vi "Post-Uninstall Custom Action.vi"(10 "Variant":variant) -> (0 "error out":errorcluster)   [LabVIEW 2020]
uses:
  <resource>/dialog/lvconfig.llb/LV Config Read String.vi
  <vilib>/Utility/config.llb/Read Key (String).vi
  <vilib>/Utility/config.llb/Read Key (I32).vi
  <resource>/dialog/lvconfig.llb/LV Config Write String.vi
  <resource>/dialog/lvconfig.llb/LV Config Write Numeric (I32).vi
  <vilib>/Utility/config.llb/NI_LVConfig.lvlib
  <vilib>/zip/NI_Unzip.lvlib
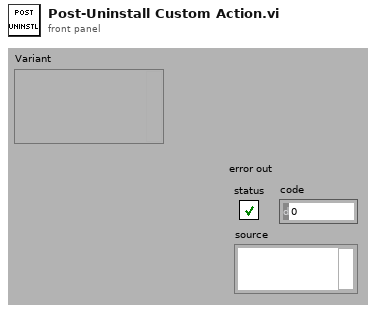
[diagram p1: front panel]
types:
  T1 = typedef "NI_LVConfig.lvlib/Config Data RefNum.ctl" = refnum<k1>
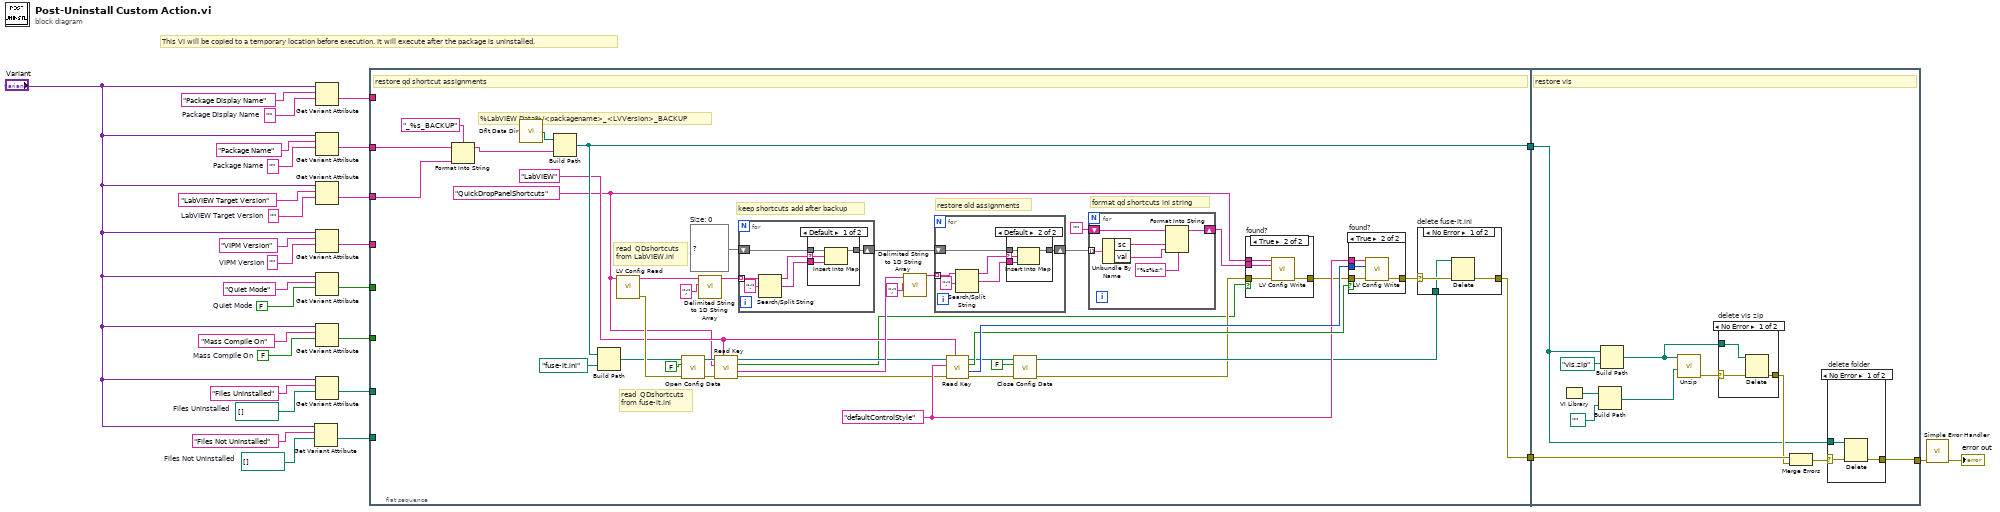
[diagram p0: block diagram]
diagram:
  w5 = path[] []  # Files Not Uninstalled
  w6 = path[] []  # Files Uninstalled
  w12 = FALSE  # Mass Compile On
  w13 = ""  # Package Display Name
  w20 = FALSE  # Quiet Mode
  w23 = ""  # VIPM Version
  w25 = ""  # LabVIEW Target Version
  w27 = ""  # Package Name
  # "This VI will be copied to a temporary location before execution. It will execute after the package is uninstalled."
  n1 = Get Variant Attribute(Variant="Variant", name="Files Not Uninstalled", default value (empty Variant)=w5) -> (value=w10:path[])  [unwired: 1 in, 3 out]
  n2 = Get Variant Attribute(Variant="Variant", name="Package Display Name", default value (empty Variant)=w13) -> (value=w19:string)  [unwired: 1 in, 3 out]
  n3 = Get Variant Attribute(Variant="Variant", name="Package Name", default value (empty Variant)=w27) -> (value=w18:string)  [unwired: 1 in, 3 out]
  n4 = Get Variant Attribute(Variant="Variant", name="LabVIEW Target Version", default value (empty Variant)=w25) -> (value=w17:string)  [unwired: 1 in, 3 out]
  n5 = Get Variant Attribute(Variant="Variant", name="VIPM Version", default value (empty Variant)=w23) -> (value=w16:string)  [unwired: 1 in, 3 out]
  n6 = Get Variant Attribute(Variant="Variant", name="Quiet Mode", default value (empty Variant)=w20) -> (value=w15:bool)  [unwired: 1 in, 3 out]
  n7 = Get Variant Attribute(Variant="Variant", name="Mass Compile On", default value (empty Variant)=w12) -> (value=w14:bool)  [unwired: 1 in, 3 out]
  n8 = Get Variant Attribute(Variant="Variant", name="Files Uninstalled", default value (empty Variant)=w6) -> (value=w9:path[])  [unwired: 1 in, 3 out]
  n9 = flat-sequence {
    tunnel: w19 -> [_]
    tunnel: w18 -> [w32]
    tunnel: w17 -> [w31]
    tunnel: w16 -> [_]
    tunnel: w15 -> [_]
    tunnel: w14 -> [_]
    tunnel: w9 -> [_]
    tunnel: w10 -> [_]
    tunnel: [w65] -> w3
    tunnel: [w62] -> w2
    tunnel: [w114] -> w4
    tunnel: w3 -> [w121]
    tunnel: w2 -> [w111]
    frame #0 {
      w56 = map{string, string} {}  # Size: 0
      w61 = "defaultControlStyle" ("key")
      w42 = "LabVIEW" ("section")
      w39 = "QuickDropPanelShortcuts" ("key")
      # "restore old assignments"
      # "format qd shortcuts ini string"
      # "read  QDshortcuts\nfrom fuse-it.ini"
      # "read  QDshortcuts\nfrom LabVIEW.ini"
      # "keep shortcuts add after backup"
      # "%LabVIEW Data%/<packagename>_<LVVersion>_BACKUP"
      # "restore qd shortcut assignments"
      n10 = Format Into String(format string="_%s_BACKUP", initial string=w32, w31) -> (resulting string=w30:string)  [unwired: 1 in, 1 out]
      n11 = call <vilib>:"Dflt Data Dir.vi"() -> ("App:Default Data Directory"=w68:path)
      n12 = Build Path(base path=w68, name or relative path=w30) -> (appended path=w62:path)
      n13 = Build Path(base path=w62, name or relative path=path "fuse-it.ini") -> (appended path=w41:path)
      n14 = call-poly <resource>:"LV Config Read.vi"("key"=w39) -> ("error out"=w46:errorcluster, "value"=w55:string)  [unwired: 4 in, 1 out]
      n15 = call <vilib>:"Open Config Data.vi"("error in (no error)"=w46, "create file if necessary (T)"=FALSE, "configuration file path"=w41) -> ("error out"=w48:errorcluster, "refnum"=w47:T1)  [unwired: 6 in, 1 out]
      n16 = call <vilib>:"Delimited String to 1D String Array.vi"("delimiter"=";", "delimited string"=w55) -> ("string array"=w57:string[])  [unwired: 9 in]
      n17 = call-poly <vilib>:"Read Key.vi"("section"=w42, "error in (no error)"=w48, "key"=w39, "refnum"=w47) -> ("error out"=w43:errorcluster, "value"=w45:string, "found?"=w36:bool, "refnum out"=w44:T1)  [unwired: 4 in]
      n18 = for {
        tunnel: w57 -> [w78] mode=indexing
        shift-right: [w76] -> w53
        shift-left: w56 -> [w77]
        n19 = Search/Split String(string=w78, search string/char (-)=":") -> (substring before match=w75:string, match + rest of string=w74:string)  [unwired: 1 in, 1 out]
        n20 = case shown="Default" w75 {
          selector: w75 -> [w81 _]
          tunnel: w77 -> [w83 w84]
          tunnel: [w82 w84] -> w76
          tunnel: w74 -> [w80 _]
          frame Default {
            n21 = Insert Into Map(map in=w83, key=w81, value=w80) -> (map out=w82:map{string, string})  [unwired: 2 out]
          }
          frame "" {
          }
        }
      }
      n22 = call <vilib>:"Delimited String to 1D String Array.vi"("delimiter"=";", "delimited string"=w45) -> ("string array"=w52:string[])  [unwired: 9 in]
      n23 = for {
        shift-right: [w90] -> w50
        shift-left: w53 -> [w89]
        tunnel: w52 -> [w87] mode=indexing
        n24 = Search/Split String(string=w87, search string/char (-)=":") -> (substring before match=w86:string, match + rest of string=w85:string)  [unwired: 1 in, 1 out]
        n25 = case shown="Default" w86 {
          selector: w86 -> [_ w93]
          tunnel: [w91 w95] -> w90
          tunnel: w89 -> [w91 w94]
          tunnel: w85 -> [_ w92]
          frame "" {
          }
          frame Default {
            n26 = Insert Into Map(map in=w94, key=w93, value=w92) -> (map out=w95:map{string, string})  [unwired: 2 out]
          }
        }
      }
      n27 = call-poly <vilib>:"Read Key.vi"("section"=w42, "error in (no error)"=w43, "key"=w61, "refnum"=w44) -> ("error out"=w60:errorcluster, "value"=w67:i32, "found?"=w66:bool, "refnum out"=w64:T1)  [unwired: 4 in]
      n28 = call <vilib>:"Close Config Data.vi"("error in (no error)"=w60, "write file if changed (T)"=FALSE, "refnum"=w64) -> ("error out"=w37:errorcluster, "file path"=w40:path)  [unwired: 7 in]
      n29 = for {
        tunnel: w50 -> [w101] mode=indexing
        shift-right: [w96] -> w38
        shift-left: "" -> [w99]
        n30 = Unbundle By Name(w101) -> ("sc"=w98:string, "val"=w97:string)
        n31 = Format Into String(format string="%s%s;", initial string=w99, w98, w97) -> (resulting string=w96:string)  [unwired: 1 in, 1 out]
      }
      n32 = case "found?" shown="True" w36 {
        tunnel: w39 -> [_ w71]
        tunnel: [w69 w72] -> w35
        tunnel: w37 -> [w69 w73]
        tunnel: w38 -> [_ w70]
        frame False {
        }
        frame True {
          n33 = call-poly <resource>:"LV Config Write.vi"("error in (no error)"=w73, "value"=w70, "key"=w71) -> ("error out"=w72:errorcluster)  [unwired: 4 in]
        }
      }
      n34 = case "found?" shown="True" w66 {
        tunnel: w35 -> [w102 w106]
        tunnel: [w102 w105] -> w34
        tunnel: w67 -> [_ w103]
        tunnel: w61 -> [_ w104]
        frame False {
        }
        frame True {
          n35 = call-poly <resource>:"LV Config Write.vi"("error in (no error)"=w106, "value"=w103, "key"=w104) -> ("error out"=w105:errorcluster)  [unwired: 4 in]
        }
      }
      n36 = case "delete fuse-it.ini" shown="No Error" w34 {
        selector: w34 -> [w109 w110]
        tunnel: w40 -> [w108 _]
        tunnel: [w107 w110] -> w65
        frame No Error {
          n37 = Delete(path (use dialog)=w108, error in=w109) -> (error out=w107:errorcluster)  [unwired: 3 in, 2 out]
        }
        frame Error {
        }
      }
    }
    frame #1 {
      # "restore vis"
      n38 = VI Library() -> (path=w118:path)
      n39 = Build Path(base path=w118, name or relative path=path "..") -> (appended path=w119:path)
      n40 = Build Path(base path=w111, name or relative path=path "vis.zip") -> (appended path=w112:path)
      n41 = call <vilib>:"Unzip.vi"("Target directory (same as Zip file if empty)"=w119, "Zip file"=w112) -> ("error out"=w117:errorcluster)  [unwired: 7 in, 2 out]
      n42 = case "delete vis zip" shown="No Error" w117 {
        selector: w117 -> [w124 w125]
        tunnel: w112 -> [w123 _]
        tunnel: [w122 w125] -> w116
        frame No Error {
          n43 = Delete(path (use dialog)=w123, error in=w124) -> (error out=w122:errorcluster)  [unwired: 3 in, 2 out]
        }
        frame Error {
        }
      }
      n44 = Merge Errors(w121, w116) -> (w115:errorcluster)
      n45 = case "delete folder" shown="No Error" w115 {
        selector: w115 -> [w128 w129]
        tunnel: w111 -> [w127 _]
        tunnel: [w126 w129] -> w114
        frame No Error {
          n46 = Delete(path (use dialog)=w127, error in=w128) -> (error out=w126:errorcluster)  [unwired: 3 in, 2 out]
        }
        frame Error {
        }
      }
    }
  }
  n47 = call <vilib>:"Simple Error Handler.vi"("error in (no error)"=w4) -> ("error out"=→"error out":errorcluster)  [unwired: 4 in, 4 out]
